vi "Scoring Intake Controls.vi"(9 "Griddy Data":T1, 10 "Reset?":bool, 11 "Operator Buttons":bool[](array[boolean])) -> (2 "Lower Cascade?":bool, 3 "Is Idle?":bool)   [LabVIEW 2020]
uses:
  manipulator/Implementation/Typedefs/Teleop Manipulator Commands.ctl
  <vilib>/Rock Robotics/WPI/Joystick/XBox Buttons Indexer.ctl
  intake sub/Implementation/intake sub Operations.ctl
  intake sub/Implementation/Typedef/intake typedef.ctl
  08a93382-5b19-475a-b453-870637c21988.vi
  <vilib>/Rock Robotics/Network Tables/NT Read Number.vi
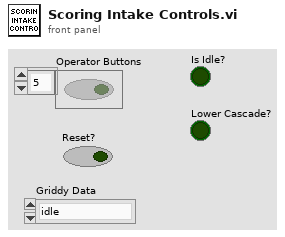
[diagram p1: front panel]
types:
  T1 = typedef "Teleop Manipulator Commands.ctl" = enum16{"idle", "intake cone sideways", "intake cone upright", "intake cone feeder", "intake cube feeder", "intake cube", "score low cone", "score low cube", "score mid cone", "score mid cube", "score high cone", "score high cube", "score mid cone up"}
  T2 = typedef "intake sub Operations.ctl" = enum16{"Reserve", "Read Current", "Immediate"}
  T3 = typedef "intake typedef.ctl" = enum16{"Intake Cone Sideways", "Intake Cone Upright", "Intake Cube", "Outtake/Score", "Shoot"}
  T4 = typedef "XBox Buttons Indexer.ctl" = enum16{"A", "B", "X", "Y", "Left Bumper", "Right Bumper", "Back", "Start", "Left Joystick", "Right Joystick"}
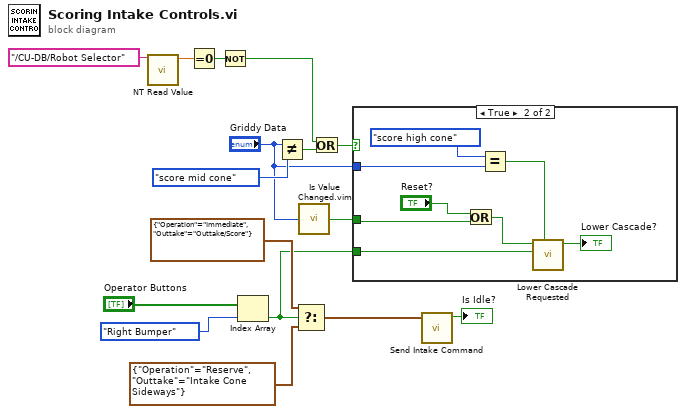
[diagram p0: block diagram]
diagram:
  n1 = call-poly <vilib>:"NT Read Value.vi"("name"="/CU-DB/Robot Selector") -> ("value"=w5:dbl)  [unwired: 8 in, 2 out]
  n2 = Equal To 0?(x=w5) -> (x = 0?=w2:bool)
  n3 = Not(x=w2) -> (.not. x?=w1:bool)
  n4 = Index Array(array="Operator Buttons", index=XBox_Buttons_Indexer."Right Bumper" ("XBox Buttons")) -> (element=w10:bool)
  n5 = Not Equal?(x="Griddy Data", y=Teleop_Manipulator_Commands."score mid cone") -> (x != y?=w4:bool)
  n6 = Select(t=cluster{"Operation":T2, "Outtake":T3} {"Operation"=enum."Immediate", "Outtake"=enum."Outtake/Score"} ("Intake Command"), s=w10, f=cluster{"Operation":T2, "Outtake":T3} {"Operation"=enum."Reserve", "Outtake"=enum."Intake Cone Sideways"}) -> (s? t:f=w11:cluster{"Operation":T2, "Outtake":T3})
  n7 = call "Is Value Changed.vim"("value"="Griddy Data") -> ("changed or first call?"=w8:bool)
  n8 = Or(x=w1, y=w4) -> (x .or. y?=w3:bool)
  n9 = case shown="True" w3 {
    tunnel: w10 -> [_ w24]
    tunnel: w8 -> [_ w21]
    tunnel: "Griddy Data" -> [_ w19]
    frame False {
    }
    frame True {
      n10 = Or(x="Reset?", y=w21) -> (x .or. y?=w22:bool)
      n11 = Equal?(x=Teleop_Manipulator_Commands."score high cone", y=w19) -> (x = y?=w17:bool)
      n12 = call "Lower Cascade Requested.vi"("Delay?"=w17, "Score Requested?"=w24, "Reset?"=w22) -> ("Lower Cascade?"=→"Lower Cascade?":bool)  [unwired: 8 in]
    }
  }
  n13 = call "Send Intake Command.vi"("Intake Command"=w11) -> ("Is Idle?"=→"Is Idle?":bool)  [unwired: 10 in]
